vi "Configure V7X.vi"(0 "VISA resource name":refnum<visa-resource-name>, 1 "START Configuration":i32, 2 "BEEP Configuration":i32, 3 "IREND Configuration":i32, 4 "FREQ Input":string="60", 5 "ARC Input":string="0", 6 "RAMPDOWN":bool=TRUE, 7 "error in (no error)":errorcluster, 8 "DIO Configuration":i32, 9 "CONTFAIL":bool=TRUE, 11 "LOCKOUT":bool=TRUE) -> (20 "VISA resource name out":refnum<visa-resource-name>, 25 "Error Message":string, 26 "Error Code":i32, 27 "error out":errorcluster)   [LabVIEW 2010, in "VITREK V7X.lvlib"]
doc: "Configures the <b>V7X</b>.\n\n<b>Note:</b> please refer to the instrument manual for the <b>Configuration Settings</b> command specifications."
uses:
  VITREK V7X.lvlib
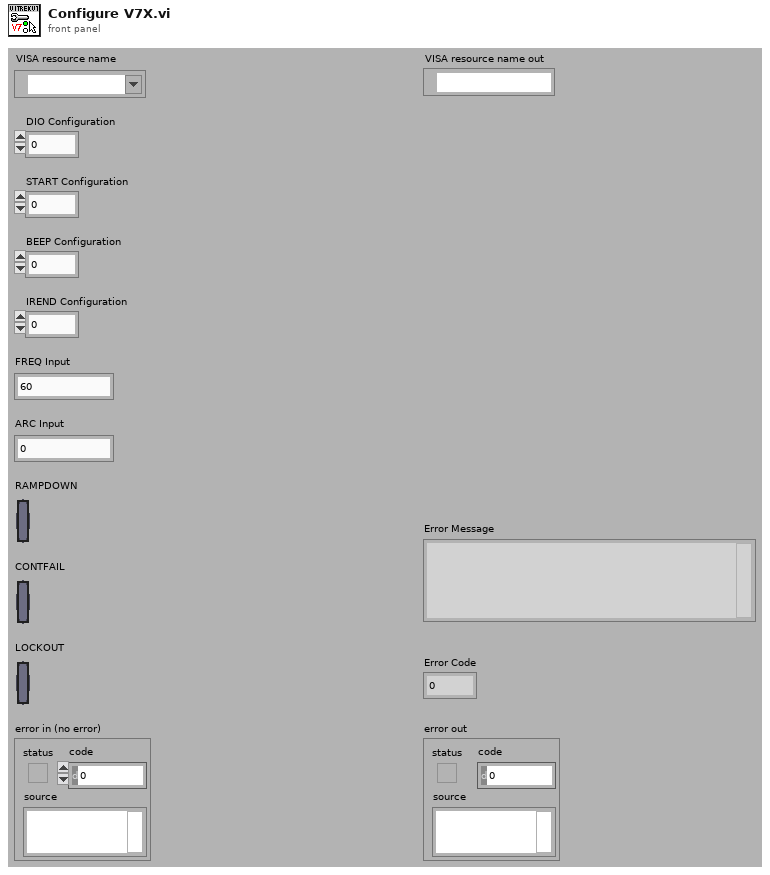
[diagram p1: front panel]
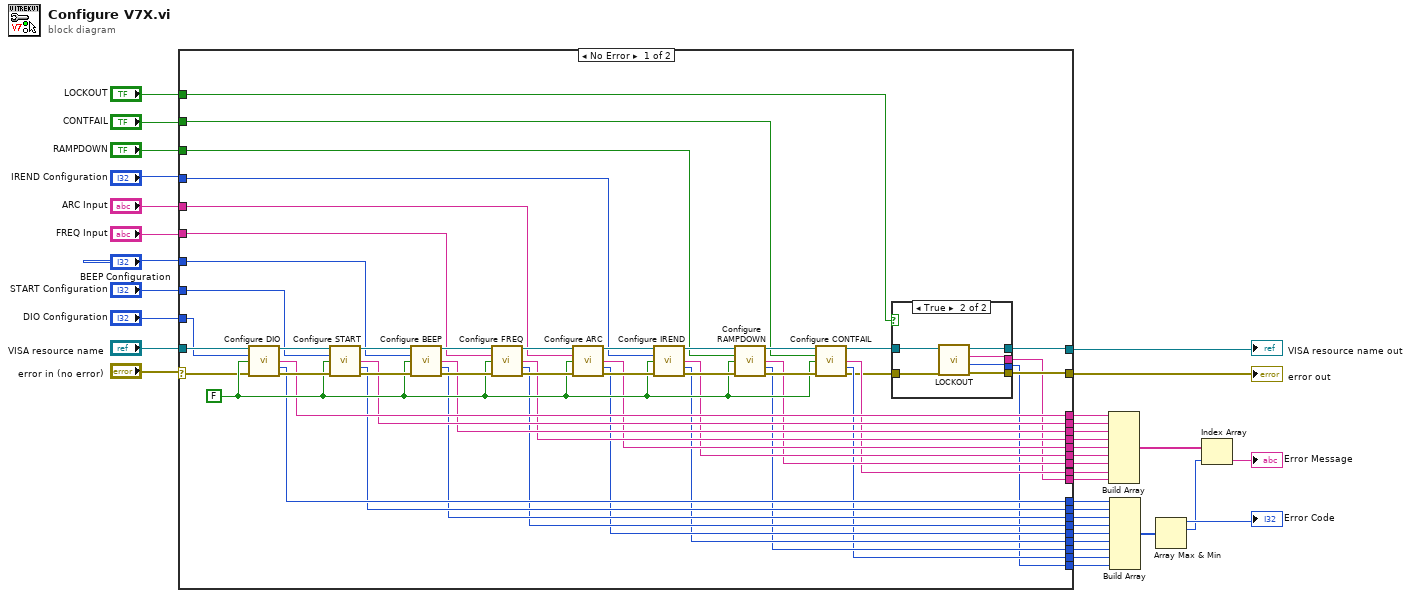
[diagram p0: block diagram]
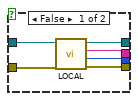
[diagram p2: hidden frame]
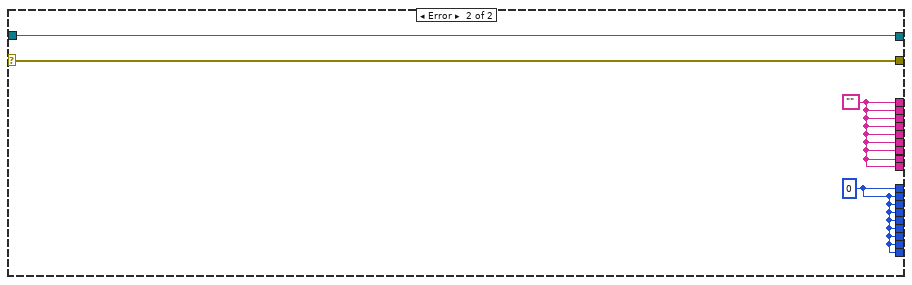
[diagram p3: hidden frame]
diagram:
  n1 = case shown="No Error" "error in (no error)" {
    selector: "error in (no error)" -> [w64 w99]
    tunnel: "VISA resource name" -> [w84 w100]
    tunnel: "START Configuration" -> [w39 _]
    tunnel: "BEEP Configuration" -> [w38 _]
    tunnel: "FREQ Input" -> [w77 _]
    tunnel: "ARC Input" -> [w74 _]
    tunnel: "IREND Configuration" -> [w37 _]
    tunnel: "RAMPDOWN" -> [w69 _]
    tunnel: "CONTFAIL" -> [w65 _]
    tunnel: [w44 w99] -> w30
    tunnel: [w46 w100] -> w29
    tunnel: [w63 w97] -> w28
    tunnel: [w62 w97] -> w27
    tunnel: [w61 w97] -> w26
    tunnel: [w60 w97] -> w25
    tunnel: [w59 w97] -> w24
    tunnel: [w58 w97] -> w23
    tunnel: [w57 w97] -> w22
    tunnel: [w56 w97] -> w21
    tunnel: [w55 w98] -> w20
    tunnel: [w54 w98] -> w19
    tunnel: [w53 w98] -> w18
    tunnel: [w52 w98] -> w17
    tunnel: [w51 w98] -> w16
    tunnel: [w50 w98] -> w15
    tunnel: [w49 w98] -> w14
    tunnel: [w48 w98] -> w13
    tunnel: "LOCKOUT" -> [w43 _]
    tunnel: [w42 w98] -> w7
    tunnel: [w41 w97] -> w6
    tunnel: "DIO Configuration" -> [w40 _]
    frame No Error {
      w66 = FALSE
      n2 = call "Configure DIO.vi"("VISA resource name"=w84, "DIO Configuration"=w40, "Configuration Query"=w66, "error in (no error)"=w64) -> ("VISA resource name out"=w83:refnum<visa-resource-name>, "Error Message"=w63:string, "Error Code"=w55:i32, "error out"=w82:errorcluster)  [unwired: 7 in, 1 out]
      n3 = call "Configure START.vi"("VISA resource name"=w83, "START Configuration"=w39, "Configuration Query"=w66, "error in (no error)"=w82) -> ("VISA resource name out"=w80:refnum<visa-resource-name>, "Error Message"=w62:string, "Error Code"=w54:i32, "error out"=w81:errorcluster)  [unwired: 7 in, 1 out]
      n4 = call "Configure BEEP.vi"("VISA resource name"=w80, "BEEP Configuration"=w38, "Configuration Query"=w66, "error in (no error)"=w81) -> ("VISA resource name out"=w78:refnum<visa-resource-name>, "Error Message"=w61:string, "Error Code"=w53:i32, "error out"=w79:errorcluster)  [unwired: 7 in, 1 out]
      n5 = call "Configure FREQ.vi"("VISA resource name"=w78, "FREQ Input"=w77, "Configuration Query"=w66, "error in (no error)"=w79) -> ("VISA resource name out"=w75:refnum<visa-resource-name>, "Error Message"=w60:string, "Error Code"=w52:i32, "error out"=w76:errorcluster)  [unwired: 7 in, 1 out]
      n6 = call "Configure ARC.vi"("VISA resource name"=w75, "ARC Input"=w74, "Configuration Query"=w66, "error in (no error)"=w76) -> ("VISA resource name out"=w73:refnum<visa-resource-name>, "Error Message"=w59:string, "Error Code"=w51:i32, "error out"=w72:errorcluster)  [unwired: 7 in, 1 out]
      n7 = call "Configure IREND.vi"("VISA resource name"=w73, "IREND Configuration"=w37, "Configuration Query"=w66, "error in (no error)"=w72) -> ("VISA resource name out"=w70:refnum<visa-resource-name>, "Error Message"=w58:string, "Error Code"=w50:i32, "error out"=w71:errorcluster)  [unwired: 7 in, 1 out]
      n8 = call "Configure RAMPDOWN.vi"("VISA resource name"=w70, "RAMPDOWN"=w69, "Configuration Query"=w66, "error in (no error)"=w71) -> ("VISA resource name out"=w67:refnum<visa-resource-name>, "Error Message"=w57:string, "Error Code"=w49:i32, "error out"=w68:errorcluster)  [unwired: 7 in, 1 out]
      n9 = call "Configure CONTFAIL.vi"("VISA resource name"=w67, "CONTFAIL"=w65, "Configuration Query"=w66, "error in (no error)"=w68) -> ("VISA resource name out"=w47:refnum<visa-resource-name>, "Error Message"=w56:string, "Error Code"=w48:i32, "error out"=w45:errorcluster)  [unwired: 7 in, 1 out]
      n10 = case shown="True" w43 {
        tunnel: w47 -> [w90 w96]
        tunnel: [w89 w95] -> w46
        tunnel: w45 -> [w88 w94]
        tunnel: [w87 w93] -> w44
        tunnel: [w85 w92] -> w42
        tunnel: [w86 w91] -> w41
        frame False {
          n11 = call "LOCAL.vi"("error in (no error)"=w88, "VISA resource name"=w90) -> ("error out"=w87:errorcluster, "Error Code"=w85:i32, "Error Message"=w86:string, "VISA resource name out"=w89:refnum<visa-resource-name>)  [unwired: 6 in]
        }
        frame True {
          n12 = call "LOCKOUT.vi"("error in (no error)"=w94, "VISA resource name"=w96) -> ("error out"=w93:errorcluster, "Error Code"=w92:i32, "Error Message"=w91:string, "VISA resource name out"=w95:refnum<visa-resource-name>)  [unwired: 6 in]
        }
      }
    }
    frame Error {
      w98 = 0 ("Error Code")
      w97 = ""
    }
  }
  "VISA resource name out" <- w29
  "error out" <- w30
  n13 = Build Array(w28, w27, w26, w25, w24, w23, w22, w21, w6) -> (w12:string[])
  n14 = Build Array(w20, w19, w18, w17, w16, w15, w14, w13, w7) -> (w11:i32[])
  n15 = Array Max & Min(array=w11) -> (max value=→"Error Code":i32, max index (indices)=w8:i32)  [unwired: 2 out]
  n16 = Index Array(array=w12, index=w8) -> (element=→"Error Message":string)
